vi "clLabview_BDPW.vi"(0 "vi_lib.lvlib:clLabview.lvclass":refnum<class "clLabview.lvclass">) -> (11 "vi_lib.lvlib:clLabview.lvclass [Out]":refnum<class "clLabview.lvclass">, 12 "Salt":string, 13 "Salt (Hex)":string, 14 "MD5 password":string, 15 "MD5-Hash 1":string, 16 "MD5-Hash 2":string, 17 "MD5 password (Hex)":string, 18 "MD5-Hash 1  (Hex)":string, 19 "MD5-Hash 2  (Hex)":string)   [LabVIEW 2011, in "vi_lib.lvlib" / "clLabview.lvclass"]
uses:
  clLabview.lvclass
  clLabview.lvclass/clLabview.ctl
  clFileReader/clFileReader.lvclass
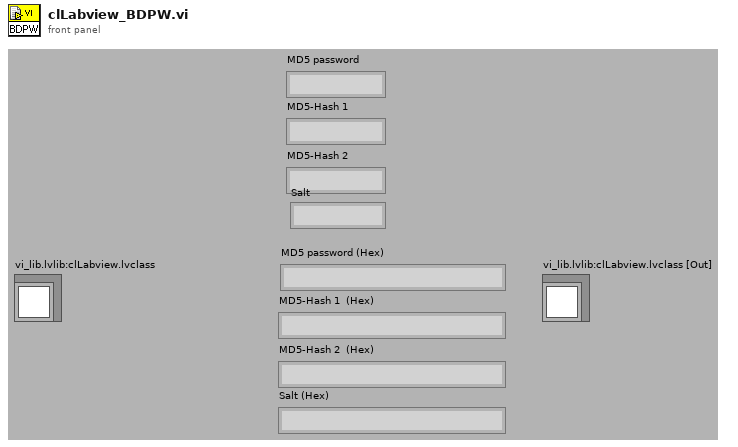
[diagram p1: front panel]
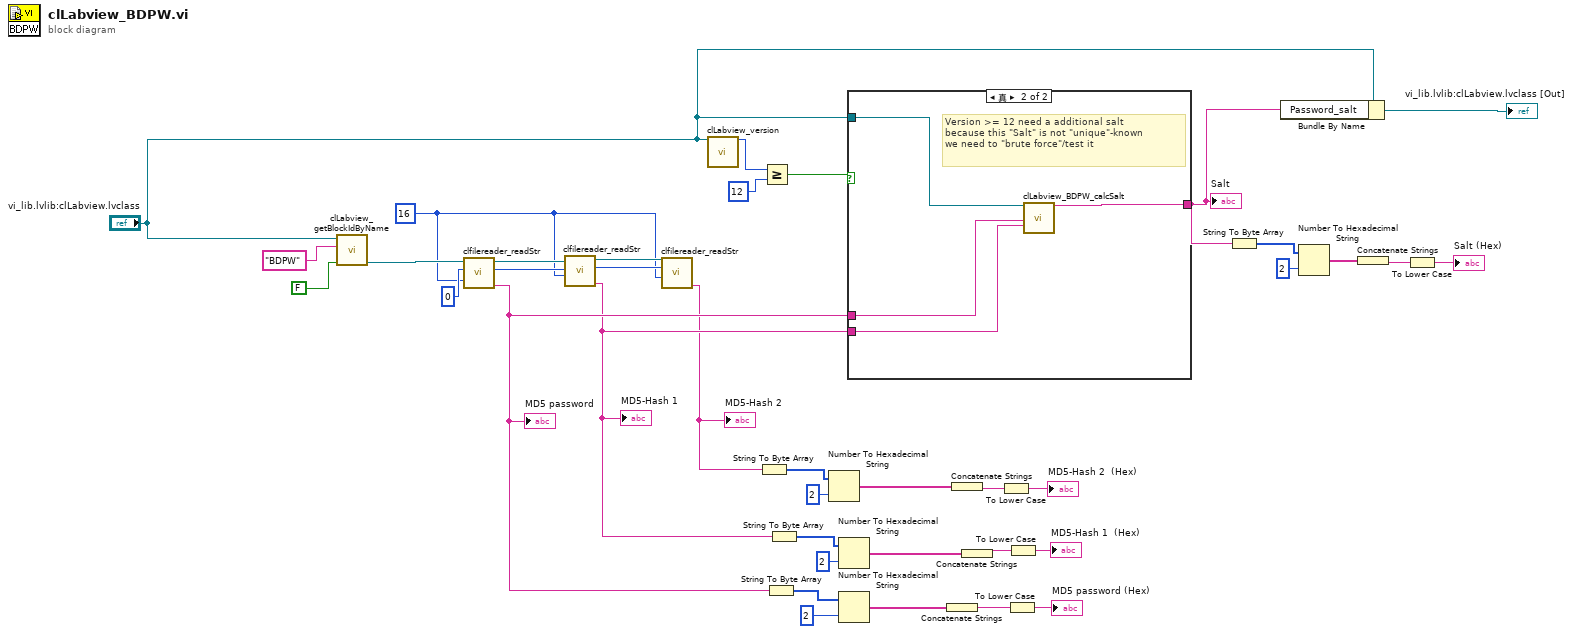
[diagram p0: block diagram]
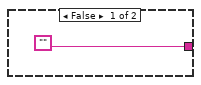
[diagram p2: hidden frame]
diagram:
  w31 = u32 16 ("size")
  n1 = call "clLabview_getBlockIdByName.vi"("use compression (off)"=FALSE, "Block Name"="BDPW", "vi_lib.lvlib:clLabview.lvclass"="vi_lib.lvlib:clLabview.lvclass") -> ("Block Content"=w37:refnum<class "clFileReader.lvclass">)  [unwired: 1 in, 6 out]
  n2 = call "clfilereader_readStr.vi"("size"=w31, "offset"=u32 0, "clFileReader.lvclass IN"=w37) -> ("ReadStr - OUT Value"=w11:string, "new offset"=w33:u32, "clFileReader.lvclass OUT"=w36:refnum<class "clFileReader.lvclass">)  [unwired: 6 out]
  "MD5 password" <- w11
  n3 = call "clfilereader_readStr.vi"("size"=w31, "offset"=w33, "clFileReader.lvclass IN"=w36) -> ("ReadStr - OUT Value"=w10:string, "new offset"=w32:u32, "clFileReader.lvclass OUT"=w35:refnum<class "clFileReader.lvclass">)  [unwired: 6 out]
  "MD5-Hash 1" <- w10
  n4 = call "clfilereader_readStr.vi"("size"=w31, "offset"=w32, "clFileReader.lvclass IN"=w35) -> ("ReadStr - OUT Value"=w9:string)  [unwired: 8 out]
  "MD5-Hash 2" <- w9
  n5 = call "clLabview_version.vi"("vi_lib.lvlib:clLabview.lvclass"="vi_lib.lvlib:clLabview.lvclass") -> ("major"=w13:u8)  [unwired: 18 out]
  n6 = String To Byte Array(string=w9) -> (unsigned byte array=w23:u8[])
  n7 = Greater Or Equal?(x=w13, y=u8 12) -> (x >= y?=w14:bool)
  n8 = String To Byte Array(string=w11) -> (unsigned byte array=w29:u8[])
  n9 = String To Byte Array(string=w10) -> (unsigned byte array=w26:u8[])
  n10 = Number To Hexadecimal String(1:i16 2 ("width (-)"), 2:w23) -> (0:w21:string[])
  n11 = Number To Hexadecimal String(1:i16 2 ("width (-)"), 2:w26) -> (0:w24:string[])
  n12 = Number To Hexadecimal String(1:i16 2 ("width (-)"), 2:w29) -> (0:w27:string[])
  n13 = case shown="真" w14 {
    tunnel: "vi_lib.lvlib:clLabview.lvclass" -> [_ w43]
    tunnel: w11 -> [_ w42]
    tunnel: w10 -> [_ w41]
    tunnel: ["" w40] -> w2
    frame False {
    }
    frame True {
      # "Version >= 12 need a additional salt\nbecause this \"Salt\" is not \"unique\"-known\nwe need to \"brute force\"/test it"
      n14 = call "clLabview_BDPW_calcSalt.vi"("vi_lib.lvlib:clLabview.lvclass"=w43, "MD5 password"=w42, "Hash 1"=w41) -> ("Salt"=w40:string)  [unwired: 1 in, 15 out]
    }
  }
  "Salt" <- w2
  n15 = Concatenate Strings(w27) -> (w16:string)
  n16 = Concatenate Strings(w21) -> (w20:string)
  n17 = Concatenate Strings(w24) -> (w17:string)
  n18 = To Lower Case(string=w20) -> (all lower case string=→"MD5-Hash 2  (Hex)":string)
  n19 = To Lower Case(string=w16) -> (all lower case string=→"MD5 password (Hex)":string)
  n20 = To Lower Case(string=w17) -> (all lower case string=→"MD5-Hash 1  (Hex)":string)
  n21 = String To Byte Array(string=w2) -> (unsigned byte array=w8:u8[])
  n22 = Bundle By Name(cluster="vi_lib.lvlib:clLabview.lvclass", "Password_salt"=w2) -> (→"vi_lib.lvlib:clLabview.lvclass [Out]":refnum<class "clLabview.lvclass">)
  n23 = Number To Hexadecimal String(1:i16 2 ("width (-)"), 2:w8) -> (0:w6:string[])
  n24 = Concatenate Strings(w6) -> (w5:string)
  n25 = To Lower Case(string=w5) -> (all lower case string=→"Salt (Hex)":string)
